vi "RW All ECAT.vi"(2 "R/W Case":T34, 7 "RT Data in":T1={"Device ref"=0, "Scan Period (uSec)"=10000, "Device Channels"={"Status"={"BD Refs"=[], "Length"=0, "FIFO Index"=0, "Data"=[]}, "Command"={"BD Refs"=[], "Data"=[], "Length"=0, "FIFO Index"=0}}, "Local Chassis"=[], "EtherCAT Masters"=[], "Async"={"Status"=refnum, "Command"=refnum, "Input FIFO"=refnum, "Input FIFO buffer"=[], "Output FIFO"=refnum, "Output FIFO buffer"=[], "Async VI Ref"=refnum}, "ECAT Reconfig"={"Reconfig Module Found"=FALSE, "VI Ref"=refnum, "Status"=refnum}, "Device Error"={"status"=FALSE, "code"=0, "source"=""}, "DeviceName"="", "PCLSync?"=FALSE} {"Device Channels"."Status"."BD Refs"."Data Reference" format="%.0x"; "Device Channels"."Command"."BD Refs"."Data Reference" format="%.0x"; "Local Chassis"."FPGA"."VS ref" format="%.0x"; "Local Chassis"."RSI Modules"."VS ref" format="%.0x"; "Local Chassis"."VS ref" format="%.0x"; "Device ref" format="%.0x"; "EtherCAT Masters"."DS402 Drive ECAT Slaves"."VS ref" format="%.0x"; "EtherCAT Masters"."REM IO ECAT Slaves"."VS ref" format="%.0x"; "EtherCAT Masters"."Generic EtherCAT Slaves"."VS ref" format="%.0x"; "EtherCAT Masters"."VS ref" format="%.0x"; "EtherCAT Masters"."EtherCAT Slaves"."FPGA"."VS ref" format="%.0x"; "EtherCAT Masters"."EtherCAT Slaves"."RSI Modules"."VS ref" format="%.0x"; "EtherCAT Masters"."EtherCAT Slaves"."VS ref" format="%.0x"}) -> (8 "RT Data out":T1={"Device ref"=0, "Scan Period (uSec)"=10000, "Device Channels"={"Status"={"BD Refs"=[], "Length"=0, "FIFO Index"=0, "Data"=[]}, "Command"={"BD Refs"=[], "Data"=[], "Length"=0, "FIFO Index"=0}}, "Local Chassis"=[], "EtherCAT Masters"=[], "Async"={"Status"=refnum, "Command"=refnum, "Input FIFO"=refnum, "Input FIFO buffer"=[], "Output FIFO"=refnum, "Output FIFO buffer"=[], "Async VI Ref"=refnum}, "ECAT Reconfig"={"Reconfig Module Found"=FALSE, "VI Ref"=refnum, "Status"=refnum}, "Device Error"={"status"=FALSE, "code"=0, "source"=""}, "DeviceName"="", "PCLSync?"=FALSE} {"Device Channels"."Status"."BD Refs"."Data Reference" format="%.0x"; "Device Channels"."Command"."BD Refs"."Data Reference" format="%.0x"; "Local Chassis"."FPGA"."VS ref" format="%.0x"; "Local Chassis"."RSI Modules"."VS ref" format="%.0x"; "Local Chassis"."VS ref" format="%.0x"; "Device ref" format="%.0x"; "EtherCAT Masters"."DS402 Drive ECAT Slaves"."VS ref" format="%.0x"; "EtherCAT Masters"."REM IO ECAT Slaves"."VS ref" format="%.0x"; "EtherCAT Masters"."Generic EtherCAT Slaves"."VS ref" format="%.0x"; "EtherCAT Masters"."VS ref" format="%.0x"; "EtherCAT Masters"."EtherCAT Slaves"."FPGA"."VS ref" format="%.0x"; "EtherCAT Masters"."EtherCAT Slaves"."RSI Modules"."VS ref" format="%.0x"; "EtherCAT Masters"."EtherCAT Slaves"."VS ref" format="%.0x"})   [LabVIEW 2016, in "Scan Engine Custom Device.lvlib"]
uses:
  Scan Engine Custom Device.lvlib
  Type Defs/RW Case.ctl
  Type Defs/RT Data.ctl
  <vilib>/NI Veristand/Custom Device API/Custom Device Item Ref.ctl
  Type Defs/Device Channels.ctl
  Type Defs/Output Data.ctl
  <vilib>/NI Veristand/Custom Device API/Block Data Reference.ctl
  <vilib>/NI Veristand/Custom Device API/Data Reference.ctl
  Type Defs/Input Data.ctl
  Type Defs/Local Chassis Data.ctl
  Type Defs/RSI Module Data.ctl
  Type Defs/Open Module IOVs.ctl
  Modules.lvlibp/RSI Module/RSI Module.lvclass
  Modules.lvlibp/RSI Module/Module Models.ctl
  Modules.lvlibp/RSI Module/Channel Type.ctl
  Type Defs/Module Config Data.ctl
  Type Defs/Mixed IO.ctl
  Type Defs/FPGA Data.ctl
  Type Defs/UDV Data.ctl
  Type Defs/UDV Data Type.ctl
  Type Defs/FXP Config.ctl
  Type Defs/Mod Size Indexes.ctl
  Type Defs/EtherCAT Master Data.ctl
  Type Defs/EtherCAT Slave Data.ctl
  Type Defs/Generic ECAT Slave RT-Data-Array.ctl
  Type Defs/Generic ECAT Slave Data Cluster.ctl
  Type Defs/Generic ECAT Slave IOV Cluster.ctl
  Type Defs/REM IO ECAT Slave RT-Data-Array.ctl
  Type Defs/REM IO ECAT Slave Data Cluster.ctl
  Type Defs/REM IO ECAT Slave IOV Cluster.ctl
  Type Defs/DS402 Drive ECAT Slave RT-Data-Array.ctl
  Type Defs/DS402 Drive ECAT Slave Data Cluster.ctl
  Type Defs/DS402 Drive ECAT Slave IOV Cluster.ctl
  Type Defs/DS402 Drive ECAT Slave Action IOV Cluster.ctl
  Type Defs/Async Data.ctl
  Type Defs/Async Status.ctl
  Type Defs/Async State.ctl
  Type Defs/Async Command.ctl
  Type Defs/ECAT Reconfig Data.ctl
  Type Defs/ECAT Reconfig Status.ctl
  Type Defs/ECAT Reconfig State.ctl
  RW Mods.vi
  RW UDVs.vi
  Read ECAT VARs.vi
  Write ECAT VARs.vi
  Read REM IO VARs.vi
  Write REM IO VARs.vi
  Read DS402 Drive VARs.vi
  Write DS402 Drive VARs.vi
  Read All Input Module Sizes.vi
  Read All Mixed Module Sizes.vi
  Write Module.vi
  Check Module Config.vi
  Read UDVs.vi
  Write UDVs.vi
  Scanned Read - UDV.vi
  <vilib>/NI Veristand/Custom Device API/NI VeriStand - Set Channel Values by Block Data Reference.vi
  Scanned Write - UDV.vi
  <vilib>/NI Veristand/Custom Device API/NI VeriStand - Get Channel Values by Block Data Reference.vi
  Read Input Modules at Indexes.vi
  Read Mixed Modules at Indexes.vi
  Scanned Write - Module.vi
  Read Input Module.vi
  Read Mixed Module.vi
  Scanned Read - Input Module.vi
  Scanned Read - Mixed Module.vi
  <vilib>/NI/syslog/Syslog Device Send.vi
  <vilib>/NI Veristand/Custom Device API/Global Data Refs.vi
  Launch Local Reconfig.vi
  DS402 StateMachine/Process DS402 SM.vi
  <vilib>/NI Veristand/Custom Device API/Custom Device API.lvlib
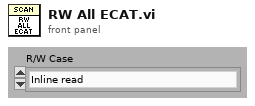
[diagram p1: front panel]
types:
  T1 = typedef "Scan Engine Custom Device.lvlib/RT Data.ctl" = cluster{"Device ref":T2, "Scan Period (uSec)":u32, "Device Channels":T3, "Local Chassis":T8[], "EtherCAT Masters":T20[], "Async":T32, "ECAT Reconfig":T33, "Device Error":errorcluster, "DeviceName":string, "PCLSync?":bool}
  T2 = typedef "Custom Device API.lvlib/Custom Device Item Ref.ctl" = u64
  T3 = typedef "Scan Engine Custom Device.lvlib/Device Channels.ctl" = cluster{"Status":T4, "Command":T7}
  T4 = typedef "Scan Engine Custom Device.lvlib/Output Data.ctl" = cluster{"BD Refs":T5[], "Length":i32, "FIFO Index":i32, "Data":dbl[]}
  T5 = typedef "Custom Device API.lvlib/Block Data Reference.ctl" = cluster{"Data Reference":T6, "Offset":u64, "Length":u64}
  T6 = typedef "Custom Device API.lvlib/Data Reference.ctl" = i32
  T7 = typedef "Scan Engine Custom Device.lvlib/Input Data.ctl" = cluster{"BD Refs":T5[], "Data":dbl[], "Length":i32, "FIFO Index":i32}
  T8 = typedef "Scan Engine Custom Device.lvlib/Local Chassis Data.ctl" = cluster{"VS ref":T2, "RSI Modules":T9[], "FPGA":T15[], "Input Mod Size Idxs":T19, "Output Modules":i32[], "MixedIO Mod Size Idxs":T19}
  T9 = typedef "Scan Engine Custom Device.lvlib/RSI Module Data.ctl" = cluster{"VS ref":T2, "IOV ref":refnum<k21>, "Open Mod refs":T10, "Module DVR":refnum<data-value>, "Slot":u32, "Model":T11, "Channel Type":T12, "EtherCAT?":bool, "CDInput Data":T7, "CDOutput Data":T4, "Module Config Data":T13, "Mixed IO":T14}
  T10 = typedef "Scan Engine Custom Device.lvlib/Open Module IOVs.ctl" = cluster{"Analog Read":refnum<k21>, "Digital Read":refnum<k21>, "Analog Write":refnum<k21>, "Digital Write":refnum<k21>}
  T11 = typedef "Modules.lvlibp/RSI Module.lvclass/Module Models.ctl" = enum16{"Empty", "NI 9201", "NI 9203", "NI 9205", "NI 9206", "NI 9207", "NI 9208", "NI 9211", "NI 9212", "NI 9213", "NI 9214", "NI 9215", "NI 9217", "NI 9219", "NI 9220", "NI 9221", "NI 9222", "NI 9223", "NI 9225", "NI 9227", "NI 9229", "NI 9233", "NI 9234", "NI 9235", "NI 9236", "NI 9237", "NI 9239", "NI 9242", "NI 9244", "NI 9263", "NI 9264", "NI 9265", "NI 9269", "NI 9375", "NI 9401", "NI 9402", "NI 9403", "NI 9411", "NI 9421", "NI 9422", "NI 9423", "NI 9425", "NI 9426", "NI 9435", "NI 9437", "NI 9472", "NI 9474", "NI 9475", "NI 9476", "NI 9477", "NI 9478", "NI 9481", "NI 9482", "NI 9485"}
  T12 = typedef "Modules.lvlibp/RSI Module.lvclass/Channel Type.ctl" = enum16{"Analog", "Digital"}
  T13 = typedef "Scan Engine Custom Device.lvlib/Module Config Data.ctl" = cluster{"Configurable?":bool, "Config Block Data Refs":T5[], "Config Data DVR":refnum<data-value>, "Previous Values":dbl[], "Local Reconfig VI Ref":refnum<vi>}
  T14 = typedef "Scan Engine Custom Device.lvlib/Mixed IO.ctl" = cluster{"Input Channel Indices":i32[], "Input Buffer":dbl[]}
  T15 = typedef "Scan Engine Custom Device.lvlib/FPGA Data.ctl" = cluster{"VS ref":T2, "IOV ref":refnum<k21>, "FPGA Target":enum16{"Local", "EtherCAT"}, "Product Code":u32, "Bitfile Signature":string, "Bitfile Path (RT)":path, "FPGA Session":u32, "Input Data":T7, "Output Data":T4, "UDVs":cluster{"From FPGA":T16[], "To FPGA":T16[]}}
  T16 = typedef "Scan Engine Custom Device.lvlib/UDV Data.ctl" = cluster{"VS ref":T2, "IOV Ref":refnum<k21>, "Name":string, "UDV Data Type":T17, "Supported Type?":bool, "FXP Config":T18, "FXP VI Ref":refnum<vi>}
  T17 = typedef "Scan Engine Custom Device.lvlib/UDV Data Type.ctl" = enum16{"Boolean", "Fixed Point", "Int8", "Int16", "Int32", "Int64", "U32 Bit Field", "UInt8", "UInt16", "UInt32", "UInt64", "Other"}
  T18 = typedef "Scan Engine Custom Device.lvlib/FXP Config.ctl" = cluster{"signed":bool, "size":u32, "integersize":i32}
  T19 = typedef "Scan Engine Custom Device.lvlib/Mod Size Indexes.ctl" = cluster{"4":i32[], "8":i32[], "16":i32[], "32":i32[], "other":i32[]}
  T20 = typedef "Scan Engine Custom Device.lvlib/EtherCAT Master Data.ctl" = cluster{"VS ref":T2, "IOV ref":refnum<k21>, "Master ID":u32, "Cyclic Data Bandwidth":u32, "EtherCAT Slaves":T21[], "Generic EtherCAT Slaves":T22, "REM IO ECAT Slaves":T25, "DS402 Drive ECAT Slaves":T28}
  T21 = typedef "Scan Engine Custom Device.lvlib/EtherCAT Slave Data.ctl" = cluster{"VS ref":T2, "IOV ref":refnum<k21>, "Position Address":u16, "RSI Modules":T9[], "FPGA":T15[], "Input Mod Size Idxs":T19, "Output Modules":i32[], "MixedIO Mod Size Idxs":T19}
  T22 = typedef "Scan Engine Custom Device.lvlib/Generic ECAT Slave RT-Data-Array.ctl" = T23[]
  T23 = typedef "Scan Engine Custom Device.lvlib/Generic ECAT Slave Data Cluster.ctl" = cluster{"VS ref":T2, "IOV ref":refnum<k21>, "Position Address":u16, "I/O Imput Vars ":T24[], "I/O Output Vars":T24[], "I/O Input Data":T7, "I/O Output Data":T4}
  T24 = typedef "Scan Engine Custom Device.lvlib/Generic ECAT Slave IOV Cluster.ctl" = cluster{"VS ref":T2, "IOV Ref":refnum<k21>, "Name":string, "UDV Data Type":T17}
  T25 = typedef "Scan Engine Custom Device.lvlib/REM IO ECAT Slave RT-Data-Array.ctl" = T26[]
  T26 = typedef "Scan Engine Custom Device.lvlib/REM IO ECAT Slave Data Cluster.ctl" = cluster{"VS ref":T2, "IOV ref":refnum<k21>, "Position Address":u16, "I/O Imput Vars ":T27[], "I/O Output Vars":T27[], "I/O Input Data":T7, "I/O Output Data":T4}
  T27 = typedef "Scan Engine Custom Device.lvlib/REM IO ECAT Slave IOV Cluster.ctl" = cluster{"VS ref":T2, "IOV Ref":refnum<k21>, "Name":string, "UDV Data Type":T17, "Scaling Factor":dbl}
  T28 = typedef "DS402 Drive ECAT Slave RT-Data-Array.ctl" = T29[]
  T29 = typedef "Scan Engine Custom Device.lvlib/DS402 Drive ECAT Slave Data Cluster.ctl" = cluster{"VS ref":T2, "IOV ref":refnum<k21>, "Position Address":u16, "I/O Input Vars ":T30[], "I/O Output Vars":T30[], "I/O Input Data":T7, "I/O Output Data":T4, "DS402 IOV":T31}
  T30 = typedef "Scan Engine Custom Device.lvlib/DS402 Drive ECAT Slave IOV Cluster.ctl" = cluster{"VS ref":T2, "IOV Ref":refnum<k21>, "Name":string, "UDV Data Type":T17, "Scaling Factor":dbl, "IOV":bool, "VS data Index":i32}
  T31 = typedef "Scan Engine Custom Device.lvlib/DS402 Drive ECAT Slave Action IOV Cluster.ctl" = cluster{"Control Word":refnum<k21>, "Status Word":refnum<k21>}
  T32 = typedef "Scan Engine Custom Device.lvlib/Async Data.ctl" = cluster{"Status":refnum<queue>, "Command":refnum<queue>, "Input FIFO":refnum<k33>, "Input FIFO buffer":dbl[], "Output FIFO":refnum<k33>, "Output FIFO buffer":dbl[], "Async VI Ref":refnum<vi>}
  T33 = typedef "Scan Engine Custom Device.lvlib/ECAT Reconfig Data.ctl" = cluster{"Reconfig Module Found":bool, "VI Ref":refnum<vi>, "Status":refnum<queue>}
  T34 = typedef "Scan Engine Custom Device.lvlib/RW Case.ctl" = enum16{"Inline read", "Inline write", "Async - Inline loop read", "Async - Inline loop write", "Async loop (read/write)"}
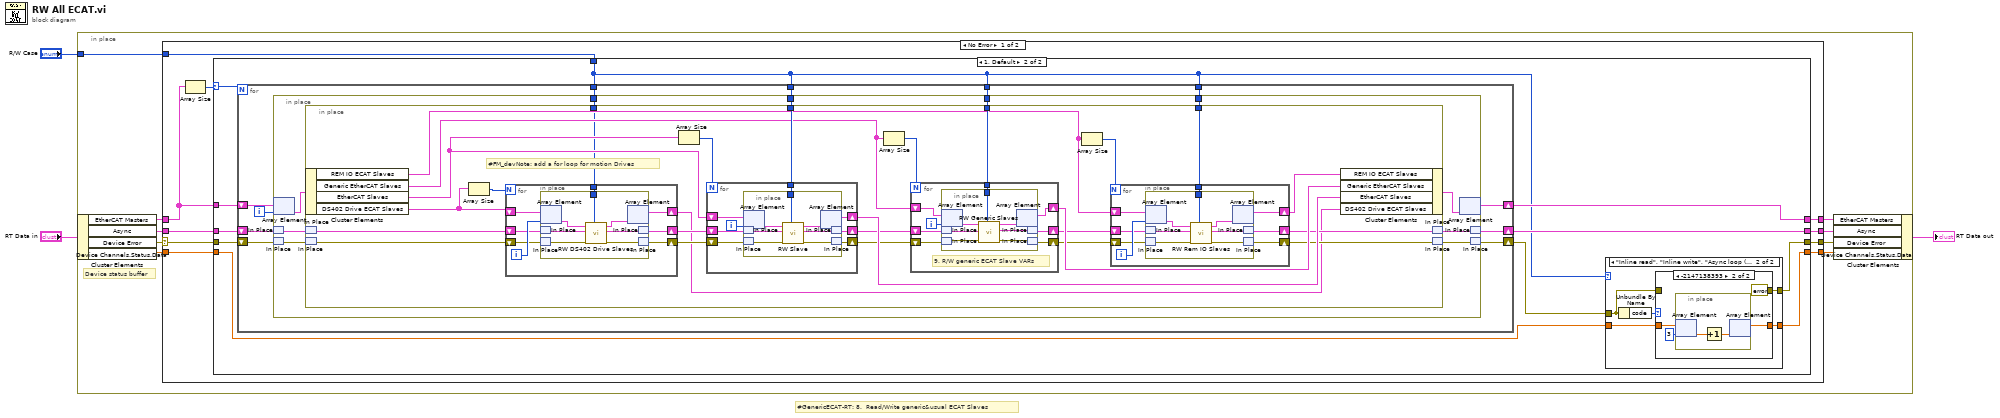
[diagram p0: block diagram]
diagram:
  # "#GenericECAT-RT: 8.  Read/Write generic&usual ECAT Slaves"
  n1 = in-place {
    in-place-border: "R/W Case" -> [w6]
    # "Device status buffer"
    n2 = in-place-cluster #1("RT Data in") -> ("EtherCAT Masters"=w7:T20[], "Async"=w9:T32, "Device Error"=w12:errorcluster, "Device Channels.Status.Data"=w5:dbl[])
    n3 = case shown="No Error" w12 {
      selector: w12 -> [w20 w163]
      tunnel: [w15 w163] -> w11
      tunnel: [w18 w162] -> w10
      tunnel: w9 -> [w21 w162]
      tunnel: [w19 w161] -> w8
      tunnel: w7 -> [w22 w161]
      tunnel: w6 -> [w17 _]
      tunnel: w5 -> [w16 w160]
      tunnel: [w13 w160] -> w4
      frame No Error {
        n4 = Array Size(array=w22) -> (size(s)=w14:i32)
        n5 = case shown="1, Default" w14 {
          selector: w14 -> [_ w30]
          tunnel: w22 -> [w26 w28]
          tunnel: w21 -> [w25 w31]
          tunnel: w20 -> [w24 w37]
          tunnel: [w26 w32] -> w19
          tunnel: [w25 w29] -> w18
          tunnel: w17 -> [_ w27]
          tunnel: w16 -> [w23 w34]
          tunnel: [w24 w35] -> w15
          tunnel: [w23 w33] -> w13
          frame 0 {
          }
          frame 1, Default {
            n6 = for {
              N: w30 -> [_]
              shift-right: [w57] -> w36
              shift-left: w37 -> [w58]
              shift-right: [w61] -> w32
              shift-left: w28 -> [w63]
              shift-right: [w59] -> w29
              shift-left: w31 -> [w60]
              tunnel: w27 -> [w56]
              tunnel: w27 -> [w55]
              tunnel: w27 -> [w54]
              tunnel: w27 -> [w53]
              i -> [w62]
              n7 = in-place {
                in-place-border: w56 -> [w67]
                in-place-border: w55 -> [w66]
                in-place-border: w54 -> [w65]
                in-place-border: w53 -> [w64]
                n8 = in-place-array #2(w63, w62) -> (w73:T20)
                n9 = in-place-match #3(w60) -> (w71:T32)
                n10 = in-place-match #4(w58) -> (w69:errorcluster)
                n11 = in-place {
                  in-place-border: w67 -> [w98]
                  in-place-border: w66 -> [w93]
                  in-place-border: w65 -> [w87]
                  in-place-border: w64 -> [w76]
                  # "#FM_devNote: add a for loop for motion Drives"
                  n12 = in-place-cluster #5(w73) -> ("REM IO ECAT Slaves"=w82:T25, "Generic EtherCAT Slaves"=w92:T22, "EtherCAT Slaves"=w97:T21[], "DS402 Drive ECAT Slaves"=w75:T28)
                  n13 = in-place-match #6(w71) -> (w81:T32)
                  n14 = in-place-match #7(w69) -> (w80:errorcluster)
                  n15 = Array Size(array=w75) -> (size(s)=w77:i32)
                  n16 = for {
                    N: w77 -> [_]
                    shift-right: [w101] -> w74
                    shift-left: w75 -> [w107]
                    shift-right: [w103] -> w79
                    shift-left: w81 -> [w105]
                    shift-right: [w102] -> w78
                    shift-left: w80 -> [w104]
                    tunnel: w76 -> [w100]
                    i -> [w106]
                    n17 = in-place {
                      in-place-border: w100 -> [w108]
                      n18 = in-place-array #8(w107, w106) -> (w110:T29)
                      n19 = in-place-match #9(w105) -> (w113:T32)
                      n20 = in-place-match #10(w104) -> (w114:errorcluster)
                      n21 = call "RW DS402 Drive Slaves.vi"("R/W Case"=w108, "error in (no error)"=w114, "Async in"=w113, "DS402 EtherCAT Slave In"=w110) -> ("error out"=w112:errorcluster, "Async out"=w111:T32, "DS402 EtherCAT Slave Out"=w109:T29)  [unwired: 5 in]
                      n22 = in-place-array #8(w109) -> (w101:T28)  [unwired: 1 out]
                      n23 = in-place-match #9(w111) -> (w103:T32)
                      n24 = in-place-match #10(w112) -> (w102:errorcluster)
                    }
                  }
                  n25 = Array Size(array=w97) -> (size(s)=w99:i32)
                  n26 = for {
                    N: w99 -> [_]
                    shift-right: [w150] -> w96
                    shift-left: w97 -> [w152]
                    shift-right: [w145] -> w94
                    shift-left: w78 -> [w146]
                    shift-right: [w148] -> w95
                    shift-left: w79 -> [w149]
                    tunnel: w98 -> [w147]
                    i -> [w151]
                    n27 = in-place {
                      in-place-border: w147 -> [w154]
                      n28 = in-place-array #11(w152, w151) -> (w153:T21)
                      n29 = in-place-match #12(w149) -> (w155:T32)
                      n30 = in-place-match #13(w146) -> (w157:errorcluster)
                      n31 = call "RW Slave.vi"("R/W Case"=w154, "error in (no error)"=w157, "Async in"=w155, "Slave in"=w153) -> ("error out"=w156:errorcluster, "Async out"=w158:T32, "Slave out"=w159:T21)  [unwired: 5 in]
                      n32 = in-place-array #11(w159) -> (w150:T21[])  [unwired: 1 out]
                      n33 = in-place-match #12(w158) -> (w148:T32)
                      n34 = in-place-match #13(w156) -> (w145:errorcluster)
                    }
                  }
                  n35 = Array Size(array=w92) -> (size(s)=w91:i32)
                  n36 = for {
                    N: w91 -> [_]
                    shift-right: [w133] -> w88
                    shift-left: w94 -> [w134]
                    shift-right: [w132] -> w89
                    shift-left: w95 -> [w135]
                    shift-right: [w136] -> w90
                    shift-left: w92 -> [w137]
                    tunnel: w93 -> [w131]
                    i -> [w130]
                    # "9. R/W generic ECAT Slave VARs"
                    n37 = in-place {
                      in-place-border: w131 -> [w142]
                      n38 = in-place-array #14(w137, w130) -> (w144:T23)
                      n39 = in-place-match #15(w135) -> (w139:T32)
                      n40 = in-place-match #16(w134) -> (w141:errorcluster)
                      n41 = call "RW Generic Slaves.vi"("R/W Case"=w142, "error in (no error)"=w141, "Async in"=w139, "Generic ECAT Slaves in"=w144) -> ("error out"=w140:errorcluster, "Async out"=w138:T32, "Generic ECAT Slaves out"=w143:T23)  [unwired: 5 in]
                      n42 = in-place-array #14(w143) -> (w136:T22)  [unwired: 1 out]
                      n43 = in-place-match #15(w138) -> (w132:T32)
                      n44 = in-place-match #16(w140) -> (w133:errorcluster)
                    }
                  }
                  n45 = Array Size(array=w82) -> (size(s)=w83:i32)
                  n46 = for {
                    N: w83 -> [_]
                    shift-right: [w116] -> w86
                    shift-left: w82 -> [w122]
                    shift-right: [w118] -> w85
                    shift-left: w89 -> [w120]
                    shift-right: [w117] -> w84
                    shift-left: w88 -> [w119]
                    tunnel: w87 -> [w115]
                    i -> [w121]
                    n47 = in-place {
                      in-place-border: w115 -> [w123]
                      n48 = in-place-array #17(w122, w121) -> (w125:T26)
                      n49 = in-place-match #18(w120) -> (w128:T32)
                      n50 = in-place-match #19(w119) -> (w129:errorcluster)
                      n51 = call "RW Rem IO Slaves.vi"("R/W Case"=w123, "error in (no error)"=w129, "Async in"=w128, "REM IO EtherCAT Slave In"=w125) -> ("error out"=w127:errorcluster, "Async out"=w126:T32, "REM IO EtherCAT Slave Out"=w124:T26)  [unwired: 5 in]
                      n52 = in-place-array #17(w124) -> (w116:T25)  [unwired: 1 out]
                      n53 = in-place-match #18(w126) -> (w118:T32)
                      n54 = in-place-match #19(w127) -> (w117:errorcluster)
                    }
                  }
                  n55 = in-place-cluster #5("REM IO ECAT Slaves"=w86, "Generic EtherCAT Slaves"=w90, "EtherCAT Slaves"=w96, "DS402 Drive ECAT Slaves"=w74) -> (w72:T20)
                  n56 = in-place-match #6(w85) -> (w70:T32)
                  n57 = in-place-match #7(w84) -> (w68:errorcluster)
                }
                n58 = in-place-array #2(w72) -> (w61:T20[])  [unwired: 1 out]
                n59 = in-place-match #3(w70) -> (w59:T32)
                n60 = in-place-match #4(w68) -> (w57:errorcluster)
              }
            }
            n61 = case shown="\"Inline read\", \"Inline write\", \"Async loop (read/write)\"" w27 {
              tunnel: w36 -> [w39 w43]
              tunnel: [w39 w42] -> w35
              tunnel: w34 -> [w38 w41]
              tunnel: [w38 w40] -> w33
              frame Default {
              }
              frame "Inline read", "Inline write", "Async loop (read/write)" {
                n62 = Unbundle By Name(w43) -> ("code"=w44:i32)
                n63 = case shown="-2147138393" w44 {
                  tunnel: w43 -> [w46 _]
                  tunnel: [w46 errorcluster {"status"=FALSE, "code"=0, "source"=""} ("error IO")] -> w42
                  tunnel: [w45 w47] -> w40
                  tunnel: w41 -> [w45 w49]
                  frame 0, Default {
                  }
                  frame -2147138393 {
                    n64 = in-place {
                      n65 = in-place-array #20(w49, 3) -> (w52:dbl)
                      n66 = Increment(x=w52) -> (x+1=w51:dbl)
                      n67 = in-place-array #20(w51) -> (w47:dbl[])  [unwired: 1 out]
                    }
                  }
                }
              }
            }
          }
        }
      }
      frame Error {
      }
    }
    n68 = in-place-cluster #1("EtherCAT Masters"=w8, "Async"=w10, "Device Error"=w11, "Device Channels.Status.Data"=w4) -> (→"RT Data out":T1)
  }
